vi "HFRR ADV v013 new software.vi"() -> ()   [LabVIEW 2025] (continued)
            n3539 = property class="DigNum (strict)"("Numeric Text.Text Colors:Text Color"="NI Text  2") -> ()  [unwired: 2 in, 2 out]
            n3540 = property class="DigNum (strict)"("Numeric Text.Text Colors:Text Color"="NI Text  2") -> ()  [unwired: 2 in, 2 out]
            n3541 = property on="Coefficient Of Friction" class="XYGraph (strict)"("Plot Area:Colors:FG Color"="GFG  2", "Plot Area:Colors:BG Color"="GBG   2") -> ()  [unwired: 2 in, 2 out]
            n3542 = property on="Humidity ( %RH )" class="XYGraph (strict)"("Plot Area:Colors:FG Color"="GFG  2", "Plot Area:Colors:BG Color"="GBG   2") -> ()  [unwired: 2 in, 2 out]
            n3543 = property on="Air Temperature  ( °C )" class="XYGraph (strict)"("Plot Area:Colors:FG Color"="GFG  2", "Plot Area:Colors:BG Color"="GBG   2") -> ()  [unwired: 2 in, 2 out]
            n3544 = property on="Sample Temperature ( °C )" class="XYGraph (strict)"("Plot Area:Colors:FG Color"="GFG  2", "Plot Area:Colors:BG Color"="GBG   2") -> ()  [unwired: 2 in, 2 out]
            n3545 = property class="DigNum (strict)"("Numeric Text.Text Colors:BG Color"="NI BG 2") -> ()  [unwired: 2 in, 2 out]
            n3546 = property class="DigNum (strict)"("Numeric Text.Text Colors:BG Color"="NI BG 2") -> ()  [unwired: 2 in, 2 out]
            n3547 = property class="DigNum (strict)"("Numeric Text.Text Colors:BG Color"="NI BG 2") -> ()  [unwired: 2 in, 2 out]
            n3548 = property class="DigNum (strict)"("Numeric Text.Text Colors:BG Color"="NI BG 2") -> ()  [unwired: 2 in, 2 out]
            n3549 = property class="DigNum (strict)"("Numeric Text.Text Colors:BG Color"="NI BG 2") -> ()  [unwired: 2 in, 2 out]
            n3550 = property class="DigNum (strict)"("Numeric Text.Text Colors:BG Color"="NI BG 2") -> ()  [unwired: 2 in, 2 out]
            n3551 = property class="DigNum (strict)"("Numeric Text.Text Colors:BG Color"="NI BG 2") -> ()  [unwired: 2 in, 2 out]
            n3552 = property class="DigNum (strict)"("Numeric Text.Text Colors:BG Color"="NI BG 2") -> ()  [unwired: 2 in, 2 out]
            n3553 = property class="DigNum (strict)"("Numeric Text.Text Colors:BG Color"="NI BG 2") -> ()  [unwired: 2 in, 2 out]
            n3554 = property class="DigNum (strict)"("Numeric Text.Text Colors:BG Color"="NI BG 2") -> ()  [unwired: 2 in, 2 out]
            n3555 = property class="DigNum (strict)"("Numeric Text.Text Colors:BG Color"="NI BG 2") -> ()  [unwired: 2 in, 2 out]
            n3556 = property class="DigNum (strict)"("Numeric Text.Text Colors:BG Color"="NI BG 2") -> ()  [unwired: 2 in, 2 out]
            n3557 = property class="DigNum (strict)"("Numeric Text.Text Colors:BG Color"="NI BG 2") -> ()  [unwired: 2 in, 2 out]
            n3558 = property class="DigNum (strict)"("Numeric Text.Text Colors:BG Color"="NI BG 2") -> ()  [unwired: 2 in, 2 out]
            n3559 = property class="DigNum (strict)"("Numeric Text.Text Colors:BG Color"="NI BG 2") -> ()  [unwired: 2 in, 2 out]
            n3560 = property class="Bool"("Colors [4]"="Boolean BC T & BG") -> ()  [unwired: 2 in, 2 out]
            n3561 = property on="Save & Continue" class="Bool (strict)"("Colors [4]"="Boolean BC T & BG") -> ()  [unwired: 2 in, 2 out]
            n3562 = property on="Heater Button" class="Bool (strict)"("Colors [4]"="Boolean BC T & BG") -> ()  [unwired: 2 in, 2 out]
            n3563 = property class="Bool"("Colors [4]"="Boolean BC T & BG") -> ()  [unwired: 2 in, 2 out]
            n3564 = property on="Humidity" class="Bool (strict)"("Colors [4]"="Boolean BC T & BG") -> ()  [unwired: 2 in, 2 out]
            n3565 = property class="Bool (strict)"("Colors [4]"="Boolean BC T & BG") -> ()  [unwired: 2 in, 2 out]
            n3566 = property on="RUN" class="Bool (strict)"("Colors [4]"="Boolean BC T & BG") -> ()  [unwired: 2 in, 2 out]
            n3567 = property on="trip1 8" class="Bool (strict)"("Colors [4]"="Boolean BC T & BG") -> ()  [unwired: 2 in, 2 out]
            n3568 = property class="Bool"("Colors [4]"="Boolean BC T & BG") -> ()  [unwired: 2 in, 2 out]
            n3569 = property class="Bool (strict)"("Colors [4]"="Boolean BC T & BG") -> ()  [unwired: 2 in, 2 out]
            n3570 = property on="OPEN 1" class="Bool (strict)"("Colors [4]"="Boolean BC T & BG 2") -> ()  [unwired: 2 in, 2 out]
            n3571 = property on="OPEN 2" class="Bool (strict)"("Colors [4]"="Boolean BC T & BG 2") -> ()  [unwired: 2 in, 2 out]
            n3572 = property on="OPEN 3" class="Bool (strict)"("Colors [4]"="Boolean BC T & BG 2") -> ()  [unwired: 2 in, 2 out]
            n3573 = property on="OPEN 4" class="Bool (strict)"("Colors [4]"="Boolean BC T & BG 2") -> ()  [unwired: 2 in, 2 out]
            n3574 = property on="OPEN" class="Bool (strict)"("Colors [4]"="Boolean BC T & BG 2") -> ()  [unwired: 2 in, 2 out]
            n3575 = property on="rstv2" class="Bool"("Colors [4]"="Boolean BC T & BG 2") -> ()  [unwired: 2 in, 2 out]
            n3576 = property on="RST CP" class="Bool"("Colors [4]"="Boolean BC T & BG 2") -> ()  [unwired: 2 in, 2 out]
            n3577 = property on="RSTV1 3" class="Bool"("Colors [4]"="Boolean BC T & BG 2") -> ()  [unwired: 2 in, 2 out]
            n3578 = property on="RSTV1 2" class="Bool"("Colors [4]"="Boolean BC T & BG 2") -> ()  [unwired: 2 in, 2 out]
          }
          frame #1 {
          }
        }
        n3579 = local read "Quit"() -> (w4455:bool)
      }
    }
    frame Enabled {
    }
  }
  n3580 = while {
    shift-right: [w4473] -> _
    shift-left: _ -> [w4474]
    shift-right: [w4471] -> _
    shift-left: T18 {"Read Heave and Surge"="", "Bytes at Heave Port"=0.0, "Heave and Surge COM Port:"="COM9", "Com Port 2"="COM7", "Residual Due"="", "Heave COM Status 2"=TRUE, "Heave COM Status"=TRUE, "Port 2"=TRUE, "Sway PPR"=6400.0, "Surge PPR"=6400.0, "Heave PPR"=6400.0, "Sway Pitch"=2.0, "Surge Pitch"=3.0, "Heave Pitch"=4.0, "Sway Pulses/mm"=320.0, "Surge Pulses/mm"=1600.0, "Heave Pulses/mm"=1600.0, "inner loop"=0.0, "Read Heave and Surge 2"="", "String 36"="", "Write S"=FALSE, "WriteCC1"=[""], "Heave COM Loop"=0, "LastCom"="", "EXIT"=FALSE, "Error Heave"={"status"=TRUE, "code"=-1073807343, "source"=""}} -> [w4470]
    shift-right: [w4468] -> _
    shift-left: enum16{"init", "MAIN", "Panel Close"}."init" -> [w4469]
    stop <- w4472 stop-if-true
    n3581 = case shown="\"MAIN\"" w4469 {
      tunnel: w4474 -> [w4488 w4503 w4564 w4566]
      tunnel: [w4482 w4512 w4564 w4566] -> w4473
      tunnel: [_ _ TRUE _] -> w4472
      tunnel: [w4478 w4509 w4562 w4565] -> w4471
      tunnel: w4470 -> [w4485 w4502 w4562 w4565]
      tunnel: [enum16{"init", "MAIN", "Panel Close"}."MAIN" w4496 _ _] -> w4468
      frame "init" {
        n3582 = Bundle By Name(cluster=w4485, "Heave and Surge COM Port:"="C3 :") -> (w4484:T18)
        n3583 = call "Instrument fgv.vi"("Enum"=T30."INIT", "error in (no error) 2"=w4488, "INPUT"=w4484) -> ("error"=w4486:errorcluster, "output"=w4481:T18)  [unwired: 6 in, 1 out]
        n3584 = case shown="Error" w4486 {
          selector: w4486 -> [w4490 _]
          tunnel: [w4490 w4494] -> w4482
          tunnel: w4481 -> [w4489 w4492]
          tunnel: [w4489 w4491] -> w4479
          frame No Error {
          }
          frame Error {
            n3585 = call "Instrument fgv.vi"("Enum"=T30."ERROR INIT", "INPUT"=w4492) -> ("error"=w4495:errorcluster, "output"=w4491:T18)  [unwired: 7 in, 1 out]
            n3586 = call <vilib>:"Clear Errors.vi"("error in (no error)"=w4495) -> ("error out"=w4494:errorcluster)  [unwired: 5 in, 1 out]
          }
        }
        n3587 = local read "LastCom"() -> (w4477:string)
        n3588 = Unbundle By Name(w4479) -> ("Heave COM Status 2"=→"COM Status" →"Instrument Status":bool, "Error Heave"=→"Error":errorcluster)  [unwired: 1 out]
        n3589 = Bundle By Name(cluster=w4479, "LastCom"=w4477) -> (w4478:T18)
      }
      frame "MAIN" {
        n3590 = Unbundle By Name(w4502) -> ("Com Port 2"=w4514:refnum<visa-resource-name>)
        n3591 = local write "Com Port 4"(w4514) -> ()
        n3592 = local read "C3 :"() -> (w4500:refnum<visa-resource-name>)
        n3593 = Bundle By Name(cluster=w4502, "Heave and Surge COM Port:"=w4500) -> (w4501:T18)
        n3594 = Equal?(x=w4514, y=w4500) -> (x = y?=w4513:bool)
        n3595 = case shown="True" w4513 {
          tunnel: [w4518 w4535] -> w4512
          tunnel: w4503 -> [w4519 w4541]
          tunnel: w4501 -> [w4517 w4539]
          tunnel: [w4516 w4534] -> w4509
          frame False {
            n3596 = call <vilib>:"Clear Errors.vi"("error in (no error)"=w4519) -> ("error out"=w4515:errorcluster)  [unwired: 5 in, 1 out]
            n3597 = call "Instrument fgv.vi"("Enum"=T30."ERROR INIT", "error in (no error) 2"=w4515, "INPUT"=w4517) -> ("error"=w4521:errorcluster, "output"=w4516:T18)  [unwired: 6 in, 1 out]
            n3598 = call <vilib>:"Clear Errors.vi"("error in (no error)"=w4521) -> ("error out"=w4518:errorcluster)  [unwired: 5 in, 1 out]
          }
          frame True {
            n3599 = call "Instrument fgv.vi"("Enum"=T30."READ", "error in (no error) 2"=w4541, "INPUT"=w4539) -> ("error"=w4540:errorcluster, "output"=w4531:T18)  [unwired: 6 in, 1 out]
            n3600 = Bundle By Name(cluster=w4531, "String 36"="String 11") -> (w4530:T18)
            n3601 = case shown="True" "Write S" {
              selector: "Write S" -> [_ w4561]
              tunnel: w4540 -> [w4554 w4560]
              tunnel: [w4554 w4559] -> w4527
              tunnel: w4530 -> [w4553 w4556]
              tunnel: [w4553 w4555] -> w4526
              frame False {
              }
              frame True {
                n3602 = Not(x=w4561) -> (.not. x?=w4557:bool)
                n3603 = local write "Write S"(w4557) -> ()
                n3604 = call "Instrument fgv.vi"("Enum"=T30."MANUAL WRITE", "error in (no error) 2"=w4560, "INPUT"=w4556) -> ("error"=w4559:errorcluster, "output"=w4555:T18)  [unwired: 6 in, 1 out]
              }
            }
            n3605 = Array Size(array="WriteHumidity") -> (size(s)=w4524:i32)
            n3606 = Greater Than 0?(x=w4524) -> (x > 0?=w4522:bool)
            n3607 = call "Instrument fgv.vi"("Enum"=T30."WRITE", "error in (no error) 2"=w4527, "WriteCC1"="WriteHumidity", "INPUT"=w4526) -> ("error"=w4537:errorcluster, "WriteCC1 2"=w4525:string[], "output"=w4536:T18)  [unwired: 5 in]
            n3608 = case shown="True" w4522 {
              tunnel: w4525 -> [_ w4543]
              frame False {
              }
              frame True {
                n3609 = local write "WriteHumidity"(w4543) -> ()
              }
            }
            n3610 = case shown="Error" w4537 {
              selector: w4537 -> [w4544 w4547]
              tunnel: w4536 -> [w4545 w4552]
              tunnel: [w4545 w4551] -> w4534
              tunnel: [w4544 w4549] -> w4535
              frame No Error {
              }
              frame Error {
                n3611 = call <vilib>:"Clear Errors.vi"("error in (no error)"=w4547) -> ("error out"=w4546:errorcluster)  [unwired: 5 in, 1 out]
                n3612 = call "Instrument fgv.vi"("Enum"=T30."ERROR INIT", "error in (no error) 2"=w4546, "INPUT"=w4552) -> ("error"=w4550:errorcluster, "output"=w4551:T18)  [unwired: 6 in, 1 out]
                n3613 = call <vilib>:"Clear Errors.vi"("error in (no error)"=w4550) -> ("error out"=w4549:errorcluster)  [unwired: 5 in, 1 out]
              }
            }
            n3614 = Unbundle By Name(w4534) -> ("LastCom"=→"LastCom":string, "Read Heave and Surge"=→"Read Humidity":string)
          }
        }
        n3615 = Unbundle By Name(w4509) -> ("Heave COM Status 2"=w4511:bool, "Heave COM Status"=w4510:bool, "Error Heave"=w4507:errorcluster, "Bytes at Heave Port"=→"Bytes at Humidity Port":dbl)
        n3616 = Unbundle By Name(w4507) -> ("status"=→"Humidity Port":bool)
        n3617 = Not(x=w4510) -> (.not. x?=w4504:bool)
        n3618 = local write "Error"(w4507) -> ()
        n3619 = Not(x=w4511) -> (.not. x?=w4505:bool)
        n3620 = local write "Instrument Status"(w4504) -> ()
        n3621 = local write "COM Status"(w4505) -> ()
        n3622 = local read "Quit"() -> (w4497:bool)
        n3623 = Select(t=enum16{"init", "MAIN", "Panel Close"}."Panel Close", s=w4497, f=enum16{"init", "MAIN", "Panel Close"}."MAIN") -> (s? t:f=w4496:enum16{"init", "MAIN", "Panel Close"})
      }
      frame "Panel Close" {
      }
      frame Default {
      }
    }
  }
  n3624 = while {
    stop <- w4592 stop-if-true
    n3625 = local read "Read Humidity"() -> (w4573:string)
    n3626 = call <vilib>:"High Resolution Polling Wait.vi"("seconds to wait"=0.1) -> ()  [unwired: 10 in, 1 out]
    n3627 = Spreadsheet String To Array(delimiter (Tab)=",", format string="", spreadsheet string=w4573, array type (2D Dbl)=string[] []) -> (array=w4587:string[])
    n3628 = for {
      tunnel: w4587 -> [w4597] mode=indexing
      tunnel: string[] ["STATE;", "SET;", "RH;", "T;", "AMB_RH;", "AMB_T;", "PUMP;", "FAN_IN;", "FAN_OUT;", "DEHUM;", "CURRENT;", "STALL;"] -> [w4596] mode=indexing
      tunnel: [w4595] -> w4586 mode=indexing
      n3629 = Match Pattern(string=w4597, regular expression=w4596) -> (after substring=w4595:string)  [unwired: 1 in, 3 out]
    }
    n3630 = Index Array(array=w4586) -> (element #1=→"STATE :":string, element #2=→"SET :":string, element #3=w4575:string, element #4=→"T :":string, element #5=w4572:string, element #6=→"AMB_T :":string, element #7=→"PUMP :":string, element #8=→"FAN_IN :":string, element #9=→"FAN_OUT :":string, element #10=→"DEHUM :":string, element #11=→"CURRENT :":string, element #12=→"STALL :":string)  [unwired: 12 in]
    "RH :" <- w4575
    "AMB_RH :" <- w4572
    n3631 = Fract/Exp String To Number(string=w4575) -> (number=w4567:dbl)  [unwired: 3 in, 1 out]
    n3632 = Fract/Exp String To Number(string=w4572) -> (number=w4571:dbl)  [unwired: 3 in, 1 out]
    n3633 = local write "Ambient Humidity :"(w4571) -> ()
    n3634 = Equal?(x=w4567, y=0.0) -> (x = y?=w4569:bool)
    n3635 = case shown="True" w4569 {
      tunnel: [w4593 w4594] -> w4568
      tunnel: w4567 -> [w4593 _]
      frame False {
        (unwired) 0.0
        "Humidity temp" <- w4593
      }
      frame True {
        n3636 = local read "Humidity temp"() -> (w4594:dbl)
      }
    }
    "RH Numeric:" <- w4568
    n3637 = local read "Quit"() -> (w4592:bool)
  }
  n3638 = disable-structure shown="Disabled" {
    frame Disabled {
      n3639 = while {
        tunnel: [w4831] -> _
        i -> [w4831]
        stop <- w4828 stop-if-true
        n3640 = local read "powstat"() -> (w4829:bool)
        n3641 = case shown="True" w4829 {
          frame False {
          }
          frame True {
            n3642 = local read "RUN"() -> (w4832:bool)
            n3643 = case shown="True" w4832 {
              frame False {
                w4862 = 65.0 ("y")
                n3644 = local read "Set Hz"() -> (w4890:dbl)
                n3645 = local read "NORMAL LOAD"() -> (w4891:dbl)
                n3646 = Multiply(x=w4890, y=60.0) -> (x*y=w4897:dbl)
                n3647 = Multiply(x=1.2 ("y"), y=0.949) -> (x*y=w4866:dbl)
                n3648 = Multiply(x=1.2 ("y"), y=0.8166) -> (x*y=w4870:dbl)
                n3649 = Multiply(x=1.2 ("y"), y=0.851) -> (x*y=w4865:dbl)
                n3650 = local read "FF 2"() -> (w4889:dbl)
                n3651 = Absolute Value(x=w4897) -> (abs(x)=w4895:dbl)
                n3652 = case shown="13.." w4889 {
                  tunnel: [1 2 3] -> w4887
                  frame 0..10, Default {
                    # "Normal"
                  }
                  frame 11, 12 {
                  }
                  frame 13.. {
                  }
                }
                "FF STATE" <- w4887
                n3653 = local read "TEMP"() -> (w4850:dbl)
                n3654 = local read item#-1() -> (w4864)
                n3655 = Less?(x=w4864, y=w4870) -> (x < y?=w4867:bool)
                n3656 = In Range and Coerce(upper limit=w4866, x=w4864, lower limit=w4865) -> (In Range?=w4868:bool)  [unwired: 1 out]
                n3657 = case shown="3601.." w4895 {
                  tunnel: [1 2 3] -> w4893
                  frame 0..3000, Default {
                    # "Normal"
                  }
                  frame 3001..3600 {
                  }
                  frame 3601.. {
                  }
                }
                n3658 = case shown="11.." w4891 {
                  tunnel: [1 3] -> w4892
                  frame 1..10, Default {
                  }
                  frame 11.. {
                  }
                }
                "NL STATE" <- w4892
                n3659 = Multiply(x=1.2 ("y"), y=0.95) -> (x*y=w4880:dbl)
                n3660 = Multiply(x=w4862, y=0.954) -> (x*y=w4854:dbl)
                n3661 = Or(x=w4867, y=w4868) -> (x .or. y?=w4869:bool)
                n3662 = Greater Or Equal?(x=w4864, y=w4880) -> (x >= y?=w4877:bool)
                n3663 = Multiply(x=w4862, y=0.99) -> (x*y=w4851:dbl)
                n3664 = Greater Or Equal?(x=w4850, y=w4851) -> (x >= y?=w4856:bool)
                n3665 = Greater Or Equal?(x=w4850, y=w4854) -> (x >= y?=w4853:bool)
                n3666 = case shown="0, 1, Default" w4864 {
                  tunnel: [1 3] -> w4881
                  frame 0, 1, Default {
                  }
                  frame 2.. {
                  }
                }
                n3667 = case shown="True" w4877 {
                  tunnel: [1 3] -> w4882
                  frame False {
                  }
                  frame True {
                  }
                }
                n3668 = case shown="True" w4869 {
                  tunnel: [1 2] -> w4883
                  frame False {
                  }
                  frame True {
                  }
                }
                n3669 = case shown="..0" w4850 {
                  tunnel: [2 3 3 1] -> w4857
                  frame 61, 62 {
                  }
                  frame 63.. {
                  }
                  frame ..0 {
                  }
                  frame 10..60, Default {
                  }
                }
                n3670 = case shown="True" w4856 {
                  tunnel: [1 3] -> w4858
                  frame False {
                  }
                  frame True {
                  }
                }
                n3671 = Number To Decimal String(number=w4893) -> (decimal integer string=w4894:string)  [unwired: 1 in]
                n3672 = case shown="True" w4853 {
                  tunnel: [1 2] -> w4859
                  frame False {
                  }
                  frame True {
                  }
                }
                n3673 = Number To Decimal String(number=1) -> (decimal integer string=→"Air temp":string)  [unwired: 1 in]
                n3674 = Number To Decimal String(number=w4887) -> (decimal integer string=→"ff_st":string)  [unwired: 1 in]
                n3675 = local write "sp_st"(w4894) -> ()
                n3676 = Number To Decimal String(number=w4892) -> (decimal integer string=→"nl_st":string)  [unwired: 1 in]
                n3677 = Build Array(w4857, w4858, w4859) -> (w4860:i32[])
                n3678 = Build Array(w4881, w4882, w4883) -> (w4884:i32[])
                n3679 = Array Max & Min(array=w4860) -> (max value=w4861:i32)  [unwired: 3 out]
                n3680 = Array Max & Min(array=w4884) -> (max value=w4885:i32)  [unwired: 3 out]
                n3681 = Number To Decimal String(number=w4861) -> (decimal integer string=w4849:string)  [unwired: 1 in]
                n3682 = Number To Decimal String(number=w4885) -> (decimal integer string=→"Stroke Ln 2":string)  [unwired: 1 in]
                n3683 = local write "temp_st"(w4849) -> ()
              }
              frame True {
                w4947 = 65.0 ("y")
                # "Healthy -1\nWarning -2\nError -3"
                n3684 = local read "TEMP"() -> (w4958:dbl)
                n3685 = local read "NORMAL LOAD"() -> (w4962:dbl)
                n3686 = local read "Set Hz"() -> (w4960:dbl)
                n3687 = Multiply(x=1.2 ("y"), y=0.949) -> (x*y=w4942:dbl)
                n3688 = Multiply(x=1.2 ("y"), y=0.8166) -> (x*y=w4938:dbl)
                n3689 = Multiply(x=1.2 ("y"), y=0.851) -> (x*y=w4943:dbl)
                n3690 = Multiply(x=w4947, y=0.954) -> (x*y=w4954:dbl)
                n3691 = Multiply(x=w4947, y=0.99) -> (x*y=w4957:dbl)
                n3692 = Greater Or Equal?(x=w4958, y=w4957) -> (x >= y?=w4952:bool)
                n3693 = Multiply(x=w4960, y=60.0) -> (x*y=w4966:dbl)
                n3694 = Greater Or Equal?(x=w4958, y=w4954) -> (x >= y?=w4955:bool)
                n3695 = local read "FF 2"() -> (w4961:dbl)
                n3696 = local read item#-1() -> (w4944)
                n3697 = Less?(x=w4944, y=w4938) -> (x < y?=w4941:bool)
                n3698 = In Range and Coerce(upper limit=w4942, x=w4944, lower limit=w4943) -> (In Range?=w4940:bool)  [unwired: 1 out]
                n3699 = Absolute Value(x=w4966) -> (abs(x)=w4964:dbl)
                n3700 = case shown="63.." w4958 {
                  tunnel: [2 3 3 1] -> w4951
                  frame 61, 62 {
                  }
                  frame 63.. {
                  }
                  frame ..0 {
                  }
                  frame 10..60, Default {
                  }
                }
                n3701 = case shown="True" w4952 {
                  tunnel: [1 3] -> w4950
                  frame False {
                  }
                  frame True {
                  }
                }
                n3702 = case shown="True" w4955 {
                  tunnel: [1 2] -> w4949
                  frame False {
                  }
                  frame True {
                  }
                }
                n3703 = Multiply(x=1.2 ("y"), y=0.95) -> (x*y=w4928:dbl)
                n3704 = case shown="1..10, Default" w4962 {
                  tunnel: [1 3] -> w4969
                  frame 1..10, Default {
                  }
                  frame 11.. {
                  }
                }
                n3705 = case shown="0..10, Default" w4961 {
                  tunnel: [1 2 3] -> w4968
                  frame 0..10, Default {
                  }
                  frame 11, 12 {
                  }
                  frame 13.. {
                  }
                }
                n3706 = case shown="3601.." w4964 {
                  tunnel: [1 2 3] -> w4963
                  frame 0..3000, Default {
                    # "Normal"
                  }
                  frame 3001..3600 {
                  }
                  frame 3601.. {
                  }
                }
                n3707 = Or(x=w4941, y=w4940) -> (x .or. y?=w4939:bool)
                n3708 = Greater Or Equal?(x=w4944, y=w4928) -> (x >= y?=w4931:bool)
                n3709 = case shown="0, 1, Default" w4944 {
                  tunnel: [1 3] -> w4927
                  frame 0, 1, Default {
                  }
                  frame 2.. {
                  }
                }
                n3710 = case shown="True" w4931 {
                  tunnel: [1 3] -> w4926
                  frame False {
                  }
                  frame True {
                  }
                }
                n3711 = case shown="True" w4939 {
                  tunnel: [1 2] -> w4925
                  frame False {
                  }
                  frame True {
                  }
                }
                n3712 = Build Array(w4951, w4950, w4949) -> (w4948:i32[])
                n3713 = Number To Decimal String(number=w4963) -> (decimal integer string=→"sp_st":string)  [unwired: 1 in]
                n3714 = Array Max & Min(array=w4948) -> (max value=w4945:i32)  [unwired: 3 out]
                "TEMP STATE" <- w4945
                n3715 = Number To Decimal String(number=w4969) -> (decimal integer string=w4972:string)  [unwired: 1 in]
                n3716 = Number To Decimal String(number=w4968) -> (decimal integer string=w4970:string)  [unwired: 1 in]
                n3717 = Number To Decimal String(number=w4945) -> (decimal integer string=→"temp_st":string)  [unwired: 1 in]
                n3718 = Build Array(w4927, w4926, w4925) -> (w4924:i32[])
                n3719 = local write "nl_st"(w4972) -> ()
                n3720 = local write "ff_st"(w4970) -> ()
                n3721 = Number To Decimal String(number=1) -> (decimal integer string=w4967:string)  [unwired: 1 in]
                n3722 = Array Max & Min(array=w4924) -> (max value=w4923:i32)  [unwired: 3 out]
                n3723 = local write "Air temp"(w4967) -> ()
                n3724 = Number To Decimal String(number=w4923) -> (decimal integer string=w4922:string)  [unwired: 1 in]
                n3725 = local write "Stroke Ln 2"(w4922) -> ()
              }
            }
            n3726 = local read "Stroke Ln 2"() -> (w4834:string)
            n3727 = local read "nl_st"() -> (w4840:string)
            n3728 = local read "ff_st"() -> (w4837:string)
            n3729 = local read "sp_st"() -> (w4838:string)
            n3730 = local read "temp_st"() -> (w4839:string)
            n3731 = local read "Air temp"() -> (w4833:string)
            n3732 = Replace Array Subset(array="in", new element #1=w4840, index #1=1 ("index"), new element #2=w4837, index #2=2 ("index"), new element #3=w4839, index #3=3 ("index"), new element #4=w4838, index #4=4 ("index"), new element #5=w4834, index #5=5 ("index"), new element #6=w4833, index #6=6 ("index"), new element #7="Sensor State" ("new element/subarray"), index #7=0 ("index")) -> (→"out":string[])
          }
        }
        n3733 = Wait (ms)(milliseconds to wait=u32 10) -> ()  [unwired: 1 out]
        n3734 = local read "Quit"() -> (w4828:bool)
      }
      n3735 = while {
        stop <- w4803 stop-if-true
        n3736 = local read "run replace"() -> (w4805:bool)
        n3737 = Wait (ms)(milliseconds to wait=u32 100) -> ()  [unwired: 1 out]
        n3738 = Equal?(x="FLAG 2", y=0.0) -> (x = y?=w4806:bool)
        n3739 = case shown="True" w4806 {
          frame False {
          }
          frame True {
            n3740 = local write "FLAG 2"(100.0 ("FLAG 2")) -> ()
            n3741 = call <vilib>:"Read Characters From File.vi"("file path (dialog if empty)"=path "C:/LAB-IQ-NXT/WO 2449 TT.sig", "convert eol? (no:F)"=FALSE ("append to file? (new file:F)")) -> ("character string"=w4809:string)  [unwired: 4 in, 3 out]
            n3742 = call <vilib>:"Read Characters From File.vi"("file path (dialog if empty)"=path "C:/LAB-IQ-NXT/WO 2449 TRH.sig", "convert eol? (no:F)"=FALSE ("append to file? (new file:F)")) -> ("character string"=w4810:string)  [unwired: 4 in, 3 out]
            n3743 = Decimal String To Number(string=w4809) -> (number=w4811:i32)  [unwired: 2 in, 1 out]
            n3744 = local write "Total No. of Tests"(w4811) -> ()
            n3745 = Decimal String To Number(string=w4810) -> (number=w4814:i32)  [unwired: 2 in, 1 out]
            n3746 = local write "SEN.RUN HRS"(w4814) -> ()
          }
        }
        n3747 = case shown="True" w4805 {
          frame False {
          }
          frame True {
            n3748 = Equal?(x="FLAG 4", y=0.0) -> (x = y?=w4818:bool)
            n3749 = case shown="False" w4818 {
              frame False {
                n3750 = Get Date/Time In Seconds() -> (seconds since 1Jan1904=w4824:timestamp)
                n3751 = local read "START 3"() -> (w4822:dbl)
                n3752 = To Double Precision Float(number=w4824) -> (double precision float=w4823:dbl)
                n3753 = Subtract(x=w4823, y=w4822) -> (x-y=→"SENSOR TIME":dbl)
              }
              frame True {
                n3754 = Get Date/Time In Seconds() -> (seconds since 1Jan1904=w4826:timestamp)
                n3755 = local write "FLAG 4"(100.0 ("FLAG")) -> ()
                n3756 = To Double Precision Float(number=w4826) -> (double precision float=→"START 3":dbl)
              }
            }
          }
        }
        n3757 = local read "Quit"() -> (w4803:bool)
      }
      n3758 = while {
        shift-right: [w4603] -> _
        shift-left: _ -> [w4604]
        tunnel: [w4599] -> _
        i -> [w4599]
        stop <- w4598 stop-if-true
        n3759 = Wait (ms)(milliseconds to wait=u32 50 ("Refresh Rate (ms)")) -> ()  [unwired: 1 out]
        n3760 = local read "Json End Flg"() -> (w4600:bool)
        n3761 = Not(x="Upld AR 2") -> ()  [unwired: 1 out]
        n3762 = local read "Upld AR 2"() -> (w4601:bool)
        n3763 = call "Elapsed Time9"("Time Target (s)"="Sen.Upload Rate (s)", "Reset"=FALSE, "Auto Reset"=TRUE) -> ("Time has Elapsed"=w4610:bool)  [unwired: 9 in, 7 out]
        n3764 = Or(x=w4610, y=w4600) -> (x .or. y?=w4606:bool)
        n3765 = case shown="True" w4606 {
          frame False {
          }
          frame True {
            w4702 = "\"SensorName\":\"" ("string")
            w4672 = " \"},{"
            w4697 = "\",\"SensorState\":\""
            w4699 = "\",\"SensorModelNumber\":\"" ("string")
            w4698 = "\",\"SensorRuntimeHours\":\"" ("string")
            n3766 = local read "model num"() -> (w4696:string[])
            n3767 = local read "Sensor name"() -> (w4715:string[])
            n3768 = local read "run"() -> (w4686:string[])
            n3769 = local read "SENSOR TIME"() -> (w4642:dbl)
            n3770 = local read "out"() -> (w4635:string[])
            n3771 = local read "Total No. of Tests"() -> (w4640:dbl)
            n3772 = Select(t=60.0, s="Run test 3", f=3600.0) -> (s? t:f=w4650:dbl)
            n3773 = Index Array(array=w4696, index #1=1 ("index")) -> (element #1=w4695:string, element #2=w4694:string, element #3=w4693:string, element #4=w4692:string, element #5=w4691:string, element #6=w4690:string)  [unwired: 5 in]
            n3774 = Index Array(array=w4686, index #1=1 ("index")) -> (element #1=w4685:string, element #2=w4684:string, element #3=w4683:string, element #4=w4682:string, element #5=w4681:string, element #6=w4680:string)  [unwired: 5 in]
            n3775 = Index Array(array=w4715, index #1=1 ("index")) -> (element #1=w4714:string, element #2=w4713:string, element #3=w4712:string, element #4=w4711:string, element #5=w4701:string, element #6=w4700:string)  [unwired: 5 in]
            n3776 = Index Array(array=w4635, index #1=1 ("index")) -> (element #1=w4667:string, element #2=w4666:string, element #3=w4665:string, element #4=w4664:string, element #5=w4663:string, element #6=w4662:string)  [unwired: 5 in]
            n3777 = local read "SEN.RUN HRS"() -> (w4638:dbl)
            n3778 = Divide(x=w4642, y=w4650) -> (x/y=w4649:dbl)
            n3779 = Increment(x=w4649) -> (x+1=w4645:dbl)
            n3780 = Number To Decimal String(number=w4645) -> (decimal integer string=→"run hrs":string)  [unwired: 1 in]
            n3781 = Divide(x=w4638, y=3600.0 ("f")) -> (x/y=w4633:dbl)
            n3782 = Round To Nearest(number=w4633) -> (nearest integer value=w4631:dbl)
            n3783 = Number To Decimal String(number=w4631) -> (decimal integer string=w4632:string)  [unwired: 1 in]
            n3784 = Number To Decimal String(number=w4640) -> (decimal integer string=w4641:string)  [unwired: 1 in]
            n3785 = local read "Model No"() -> (w4646:string)
            n3786 = local read "UUID"() -> (w4741:string)
            n3787 = local read "Serial No"() -> (w4745:string)
            n3788 = local read "Secret Key"() -> (w4746:string)
            n3789 = Concatenate Strings("\",\"MachineSerialNumber\":\"" ("string"), w4745) -> (w4749:string)
            n3790 = Concatenate Strings("\",\"ModelNumber\":\"" ("string"), w4646) -> (w4647:string)
            n3791 = Concatenate Strings("\",\"MachineRuntimeHours\":\"" ("string"), w4632) -> (w4750:string)
            n3792 = Concatenate Strings("\",\"MachineRuntimeCycles\":\"", w4641) -> (w4743:string)
            n3793 = Concatenate Strings(w4699, w4695) -> (w4729:string)
            n3794 = Concatenate Strings(w4698, w4685) -> (w4730:string)
            n3795 = Concatenate Strings(w4697, w4667) -> (w4728:string)
            n3796 = Concatenate Strings(w4749, w4647, w4750, w4743) -> (w4752:string)
            n3797 = Concatenate Strings(w4699, w4694) -> (w4726:string)
            n3798 = Concatenate Strings(w4698, w4684) -> (w4725:string)
            n3799 = Concatenate Strings(w4697, w4666) -> (w4727:string)
            n3800 = Concatenate Strings(w4699, w4693) -> (w4721:string)
            n3801 = Concatenate Strings(w4698, w4683) -> (w4722:string)
            n3802 = Concatenate Strings(w4697, w4665) -> (w4720:string)
            n3803 = Concatenate Strings(w4699, w4692) -> (w4718:string)
            n3804 = Concatenate Strings(w4698, w4682) -> (w4717:string)
            n3805 = Concatenate Strings(w4697, w4664) -> (w4719:string)
            n3806 = Concatenate Strings(w4729, w4730, w4728) -> (w4731:string)
            n3807 = Concatenate Strings(w4699, w4691) -> (w4708:string)
            n3808 = Concatenate Strings(w4698, w4681) -> (w4709:string)
            n3809 = Concatenate Strings(w4699, w4690) -> (w4705:string)
            n3810 = Concatenate Strings(w4698, w4680) -> (w4704:string)
            n3811 = Concatenate Strings(w4697, w4663) -> (w4707:string)
            n3812 = Concatenate Strings(w4697, w4662) -> (w4706:string)
            n3813 = Concatenate Strings("{\"SecretKey\":\"", w4746, w4752, "\",\"UUID\" : \"", w4741, "\",\"SensorInformation\":", "[{" ("string")) -> (w4679:string)
            n3814 = Concatenate Strings(w4726, w4725, w4727) -> (w4724:string)
            n3815 = Concatenate Strings(w4721, w4722, w4720) -> (w4723:string)
            n3816 = Concatenate Strings(w4718, w4717, w4719) -> (w4716:string)
            n3817 = Concatenate Strings(w4708, w4709, w4707) -> (w4710:string)
            n3818 = Concatenate Strings(w4705, w4704, w4706) -> (w4703:string)
            n3819 = Concatenate Strings(w4702, w4714, w4731, w4672) -> (w4678:string)
            n3820 = Concatenate Strings(w4702, w4713, w4724, w4672) -> (w4677:string)
            n3821 = Concatenate Strings(w4702, w4712, w4723, w4672) -> (w4676:string)
            n3822 = Concatenate Strings(w4702, w4711, w4716, w4672) -> (w4675:string)
            n3823 = Concatenate Strings(w4702, w4701, w4710, w4672) -> (w4674:string)
            n3824 = Concatenate Strings(w4702, w4700, w4703, "\"}" ("string")) -> (w4673:string)
            n3825 = Concatenate Strings(w4679, w4678, w4677, w4676, w4675, w4674, w4673, "]}" ("string")) -> (w4670:string)
            n3826 = local read "SEN.RUN HRS"() -> (w4637:dbl)
            n3827 = disable-structure shown="Disabled" {
              frame Disabled {
                n3828 = local read "state"() -> (w4756:string[])
                n3829 = Delete From Array(array=w4756, index=0) -> (array with subset deleted=w4754:string[])  [unwired: 1 in, 1 out]
                n3830 = for {
                  N: 6 -> [_]
                  tunnel: w4754 -> [w4767] mode=indexing
                  tunnel: [w4766] -> w4753 mode=indexing
                  n3831 = Equal?(x=w4767, y="Warning") -> (x = y?=w4763:bool)
                  n3832 = Equal?(x=w4767, y="Healthy") -> (x = y?=w4760:bool)
                  n3833 = Select(t="2" ("y"), s=w4763, f="3" ("y")) -> (s? t:f=w4758:string)
                  n3834 = Select(t="1" ("y"), s=w4760, f=w4758) -> (s? t:f=w4766:string)
                }
                "state1" <- w4753
              }
              frame Enabled {
              }
            }
            n3835 = stacked-sequence {
              tunnel: w4670 -> [w4778 _ _]
              tunnel: [_ _ w4794] -> _
              frame #0 {
                (unwired) FALSE ("convert eol (F)")
                w4780 = enum16{"start", "end", "current"}."start" ("pos mode (0:2)")
                n3836 = local read "Path"() -> (w4774:path)
                n3837 = Path To String(path=w4774) -> (string=w4786:string)
                n3838 = Concatenate Strings(w4786, "\\", "Sensor File Name") -> (w4787:string)
                n3839 = local write "standard output 2"(" ") -> ()
                n3840 = String To Path(string=w4787) -> (path=w4777:path)
                n3841 = call <vilib>:"Open_Create_Replace File.vi"("advisory dialog? (display:T)"=FALSE, "function (open:0)"=T31."create or replace", "file path"=w4777) -> ("error out"=w4790:errorcluster, "refnum"=w4789:refnum<file>)  [unwired: 5 in, 2 out]
                n3842 = Set File Position(refnum=w4789, from (0:start)=w4780, error in=w4790) -> (refnum out=w4770:refnum<file>, error out=w4769:errorcluster)  [unwired: 1 in]
                n3843 = Write to Binary File(file (use dialog)=w4770, data=" ", error in=w4769, 5:FALSE ("prepend array or string size? (T)")) -> (refnum out=w4781:refnum<file>, error out=w4782:errorcluster)  [unwired: 2 in, 1 out]
                n3844 = Set File Position(offset (in bytes) (0)=w4780, refnum=w4781, error in=w4782) -> (refnum out=w4773:refnum<file>, error out=w4772:errorcluster)  [unwired: 1 in]
                n3845 = Write to Binary File(file (use dialog)=w4773, data=w4778, error in=w4772, 5:FALSE ("prepend array or string size? (T)")) -> (error out=w4776:errorcluster)  [unwired: 2 in, 2 out]
                n3846 = flat-sequence {
                  tunnel: w4777 -> [w4792]
                  tunnel: w4776 -> [_]
                  frame #0 {
                    n3847 = call <vilib>:"Read Characters From File.vi"("file path (dialog if empty)"=w4792) -> ("character string"=→"Sensor Health JSON string":string)  [unwired: 5 in, 3 out]
                  }
                }
                "SinglePoint  2" <- w4778
              }
              frame #1 {
              }
              frame #2 {
                (unwired) "\"Stored\": true" ("string")
                n3848 = call <vilib>:"System Exec.vi"("run minimized? (F)"=TRUE, "wait until completion? (T)"=TRUE, "working directory"=path "C:/LAB-IQ-NXT", "command line"="C:\\LAB-IQ-NXT\\JPostH.bat") -> ("standard error"=→"Respose From Server 2":string, "standard output"=w4797:string)  [unwired: 4 in, 2 out]
                "standard output 2" <- w4797
                n3849 = Match Pattern(string=w4797, regular expression="JSONH Check String") -> (match substring=w4795:string, offset past match=w4794:i32)  [unwired: 1 in, 2 out]
                n3850 = Equal?(x=w4795, y="JSONH Check String") -> (x = y?=→"Upload \nConfirmed 2":bool)
              }
            }
            n3851 = Divide(x=w4637, y=3600.0 ("f")) -> (x/y=w4630:dbl)
            n3852 = local read "run time"() -> (w4687:string[])
            n3853 = Round To Nearest(number=w4630) -> (nearest integer value=w4629:dbl)
            n3854 = Number To Decimal String(number=w4629) -> (decimal integer string=w4628:string)  [unwired: 1 in]
            n3855 = Index Array(array="Sensor Information", index (col) #1=0 ("disabled index (col)"), index (col) #2=1 ("index (col)"), index (col) #3=2 ("index (col)"), index (col) #4=3 ("index (col)")) -> (element #1=→"Sensor name":string[], element #2=→"model num":string[], element #3=→"run time":string[], element #4=→"state":string[])  [unwired: 4 in]
            n3856 = Insert Into Array(array=w4687, index=1, new element #1=w4628, new element #2=w4628, new element #3=w4628, new element #4=w4628, new element #5=w4628, new element #6=w4628) -> (w4652:string[])
            "run" <- w4652
            n3857 = local read "out"() -> (w4634:string[])
            n3858 = local read "Sensor Information"() -> (w4654:string[][])
            n3859 = Replace Array Subset(array=w4654, new element #1=w4652, index (col) #1=2 ("disabled index (col)"), new element #2=w4634, index (col) #2=3 ("index (col)")) -> (w4653:string[][])  [unwired: 2 in]
            n3860 = local write "Sensor Information"(w4653) -> ()
          }
        }
        n3861 = case shown="True" w4601 {
          frame False {
          }
          frame True {
            n3862 = Equal?(x="FLAG", y=0.0) -> (x = y?=w4618:bool)
            n3863 = case shown="False" w4618 {
              frame False {
                n3864 = Get Date/Time In Seconds() -> (seconds since 1Jan1904=w4624:timestamp)
                n3865 = local read "START 2"() -> (w4622:dbl)
                n3866 = To Double Precision Float(number=w4624) -> (double precision float=w4623:dbl)
                n3867 = Subtract(x=w4623, y=w4622) -> (x-y=→"SENSOR TIME  2":dbl)
              }
              frame True {
                n3868 = Get Date/Time In Seconds() -> (seconds since 1Jan1904=w4626:timestamp)
                n3869 = To Double Precision Float(number=w4626) -> (double precision float=→"START 2":dbl)
                n3870 = local write "FLAG"(100.0 ("FLAG")) -> ()
              }
            }
          }
        }
        n3871 = disable-structure shown="Disabled" {
          disable-tunnel: w4604 -> [w4613 _]
          disable-tunnel: [w4612 _] -> w4603
          frame Disabled {
            n3872 = local read "Json St Flg"() -> (w4611:bool)
            n3873 = case shown="True" w4611 {
              tunnel: w4613 -> [w4614 w4616]
              tunnel: [w4614 w4615] -> w4612
              frame False {
              }
              frame True {
                n3874 = Increment(x=w4616) -> (x+1=w4615:dbl)
                "T cycle" <- w4615
                n3875 = local write "Json St Flg"(FALSE ("Json St Flg")) -> ()
              }
            }
          }
          frame Enabled {
          }
        }
        n3876 = local read "Quit"() -> (w4598:bool)
      }
    }
    frame Enabled {
    }
  }
  n3877 = stacked-sequence {
    tunnel: [w4996] -> w38
    frame #0 {
      w4996 = FALSE ("Upload \nConfirmed")
      n3878 = local write "Upload \nConfirmed"(w4996) -> ()
      n3879 = local write "St Str"("") -> ()
    }
  }
  n3880 = disable-structure shown="Disabled" {
    disable-tunnel: w38 -> [w4997 _]
    frame Disabled {
      n3881 = case shown="True" {
        selector: _ -> [_ _]
        tunnel: w4997 -> [_ w4998]
        frame False {
        }
        frame True {
          n3882 = while {
            tunnel: [w5004] -> _
            tunnel: w4998 -> [_]
            i -> [w5004]
            stop <- w4999 stop-if-true
            n3883 = local read "Json End Flg"() -> (w5003:bool)
            n3884 = Wait (ms)(milliseconds to wait=u32 20 ("Refresh Rate (ms)")) -> ()  [unwired: 1 out]
            n3885 = local read "refresh flag"() -> (w5000:bool)
            n3886 = local read "RUN"() -> (w5001:bool)
            n3887 = And(x=w5001, y=w5000) -> (x .and. y?=w5002:bool)
            n3888 = Or(x=w5002, y=w5003) -> (x .or. y?=w5005:bool)
            "AR Led" <- w5005
            n3889 = case shown="True" w5005 {
              frame False {
              }
              frame True {
                w5022 = "\",\""
                n3890 = local read "UUID"() -> (w5020:string)
                n3891 = local write "refresh flag"(FALSE ("refresh flag")) -> ()
                n3892 = local read "time"() -> (w5009:dbl)
                n3893 = Multiply(x=w5009, y=60.0) -> (x*y=w5008:dbl)
                n3894 = Concatenate Strings("UUID\" : \"", w5020, "\"}") -> (w5023:string)
                n3895 = Number To Fractional String(number=w5008, width (-)=i16 10, precision (6)=i16 4) -> (F-format string=w5037:string)  [unwired: 1 in]
                n3896 = Concatenate Strings("{", "\"Time\":\"", w5037, w5022) -> (w5032:string)
                n3897 = stacked-sequence {
                  tunnel: w5022 -> [w5085 w5093 w5100 w5108 w5116 w5125 w5132]
                  tunnel: [w5086 _ _ _ _ _ _] -> w5036
                  tunnel: [_ w5094 _ _ _ _ _] -> w5035
                  tunnel: [_ _ w5101 _ _ _ _] -> w5034
                  tunnel: [_ _ _ w5110 _ _ _] -> w5033
                  tunnel: w5023 -> [_ _ _ _ _ _ w5143]
                  tunnel: [_ _ _ _ _ _ w5142] -> w5019
                  tunnel: [_ _ _ _ _ w5122 _] -> w5018
                  tunnel: [_ _ _ _ w5115 _ _] -> w5017
                  frame #0 {
                    n3898 = local read "NORMAL LOAD"() -> (w5084:dbl)
                    n3899 = Number To Fractional String(number=w5084, width (-)=i16 10, precision (6)=i16 4) -> (F-format string=w5087:string)  [unwired: 1 in]
                    n3900 = Concatenate Strings("NormalLoad\":\"", w5087, w5085) -> (w5086:string)
                  }
                  frame #1 {
                    n3901 = local read "Temp"() -> (w5092:dbl)
                    n3902 = Number To Fractional String(number=w5092, width (-)=i16 10, precision (6)=i16 4) -> (F-format string=w5095:string)  [unwired: 1 in]
                    n3903 = Concatenate Strings("Temperature\":\"", w5095, w5093) -> (w5094:string)
                  }
                  frame #2 {
                    n3904 = local read "cof"() -> (w5098:dbl)
                    n3905 = Number To Fractional String(number=w5098, width (-)=i16 10, precision (6)=i16 4) -> (F-format string=w5102:string)  [unwired: 1 in]
                    n3906 = Concatenate Strings("FrictionalForce\":\"", w5102, w5100) -> (w5101:string)
                  }
                  frame #3 {
                    n3907 = local read "Set Hz"() -> (w5106:dbl)
                    n3908 = Multiply(x=w5106, y=60.0) -> (x*y=w5105:dbl)
                    n3909 = Number To Fractional String(number=w5105, width (-)=i16 10, precision (6)=i16 4) -> (F-format string=w5111:string)  [unwired: 1 in]
                    n3910 = Concatenate Strings("Speed\":\"", w5111, w5108) -> (w5110:string)
                  }
                  frame #4 {
                    n3911 = local read item#-1() -> (w5114)
                    n3912 = Number To Fractional String(number=w5114, width (-)=i16 10, precision (6)=i16 4) -> (F-format string=w5118:string)  [unwired: 1 in]
                    n3913 = Concatenate Strings("LinearDeformation\":\"", w5118, w5116) -> (w5115:string)
                  }
                  frame #5 {
                    n3914 = local read "AIR TEMP"() -> (w5121:dbl)
                    n3915 = local read "Json St Flg"() -> (w5123:bool)
                    n3916 = local read "Json End Flg"() -> (w5124:bool)
                    n3917 = Number To Fractional String(number=w5121, width (-)=i16 10, precision (6)=i16 4) -> (F-format string=w5127:string)  [unwired: 1 in]
                    n3918 = Concatenate Strings("Vibration\":\"", w5127, w5125) -> (w5122:string)
                    n3919 = And(x=w5123, y=w5124) -> ()  [unwired: 1 out]
                  }
                  frame #6 {
                    n3920 = local read "Json End Flg"() -> (w5131:bool)
                    n3921 = Get Date/Time In Seconds() -> (seconds since 1Jan1904=w5139:timestamp)
                    n3922 = local read "Json St Flg"() -> (w5130:bool)
                    n3923 = To Double Precision Float(number=w5139) -> (double precision float=w5138:dbl)
                    n3924 = Subtract(x=w5138, y=2082844800.0) -> (x-y=w5136:dbl)
                    n3925 = Number To Fractional String(number=w5136, width (-)=i16 12, precision (6)=i16 0) -> (F-format string=w5133:string)  [unwired: 1 in]
                    n3926 = case shown="True" w5131 {
                      tunnel: ["" w5146] -> w5140
                      tunnel: w5133 -> [_ w5147]
                      tunnel: w5132 -> [_ w5145]
                      frame False {
                      }
                      frame True {
                        n3927 = local write "Json End Flg"(FALSE ("Json St Flg")) -> ()
                        n3928 = Concatenate Strings("End\": \"", w5147, w5145) -> (w5146:string)
                      }
                    }
                    n3929 = case shown="True" w5130 {
                      tunnel: [w5150 w5153] -> w5141
                      tunnel: w5133 -> [_ w5154]
                      tunnel: w5132 -> [_ w5151]
                      frame False {
                        n3930 = local read "St Str"() -> (w5150:string)
                      }
                      frame True {
                        n3931 = Concatenate Strings("Start\":\"", w5154, w5151) -> (w5153:string)
                        "St Str" <- w5153
                        n3932 = local write "Json St Flg"(FALSE ("Json St Flg")) -> ()
                      }
                    }
                    n3933 = Concatenate Strings(w5141, w5140, w5143) -> (w5142:string)
                  }
                }
                n3934 = local read "FILE"() -> (w5011:string)
                n3935 = Concatenate Strings("\",\"OperatorID\":\"" ("string"), "Operator ID") -> (w5014:string)
                n3936 = Concatenate Strings("\",\"DatasetTitle\":\"" ("string"), w5011) -> (w5013:string)
                n3937 = Concatenate Strings("\",\"SerialNumber\":\"" ("string"), "Serial No") -> (w5043:string)
                n3938 = Concatenate Strings("\",\"ModelNumber\":\"" ("string"), "Model No") -> (w5042:string)
                n3939 = Concatenate Strings(w5043, w5042) -> (w5025:string)
                n3940 = Concatenate Strings("{\"SecretKey\":\"", "Secret Key", w5025, w5014, w5013, "\",\"Samples\":[") -> (w5030:string)
                n3941 = Concatenate Strings(w5032, w5036, w5035, w5034, w5033, w5017, w5018, w5019) -> (w5031:string)
                n3942 = Concatenate Strings(w5030, w5031, "]}") -> (w5029:string)
                n3943 = stacked-sequence {
                  tunnel: w5029 -> [w5058 _ _]
                  tunnel: [_ _ w5075] -> _
                  frame #0 {
                    (unwired) FALSE ("convert eol (F)")
                    w5060 = enum16{"start", "end", "current"}."start" ("pos mode (0:2)")
                    n3944 = Path To String(path="Path") -> (string=w5066:string)
                    n3945 = Concatenate Strings(w5066, "\\", "Data File Name") -> (w5068:string)
                    n3946 = local write "standard output"(" ") -> ()
                    n3947 = String To Path(string=w5068) -> (path=w5057:path)
                    n3948 = call <vilib>:"Open_Create_Replace File.vi"("advisory dialog? (display:T)"=FALSE, "function (open:0)"=T31."create or replace", "file path"=w5057) -> ("error out"=w5071:errorcluster, "refnum"=w5070:refnum<file>)  [unwired: 5 in, 2 out]
                    n3949 = Set File Position(refnum=w5070, from (0:start)=w5060, error in=w5071) -> (refnum out=w5051:refnum<file>, error out=w5050:errorcluster)  [unwired: 1 in]
                    n3950 = Write to Binary File(file (use dialog)=w5051, data=" ", error in=w5050, 5:FALSE ("prepend array or string size? (T)")) -> (refnum out=w5061:refnum<file>, error out=w5062:errorcluster)  [unwired: 2 in, 1 out]
                    n3951 = Set File Position(offset (in bytes) (0)=w5060, refnum=w5061, error in=w5062) -> (refnum out=w5054:refnum<file>, error out=w5053:errorcluster)  [unwired: 1 in]
                    n3952 = Write to Binary File(file (use dialog)=w5054, data=w5058, error in=w5053, 5:FALSE ("prepend array or string size? (T)")) -> (error out=w5056:errorcluster)  [unwired: 2 in, 2 out]
                    n3953 = flat-sequence {
                      tunnel: w5057 -> [w5073]
                      tunnel: w5056 -> [_]
                      frame #0 {
                        n3954 = call <vilib>:"Read Characters From File.vi"("file path (dialog if empty)"=w5073) -> ("character string"=→"JSON string":string)  [unwired: 5 in, 3 out]
                      }
                    }
                    "SinglePoint" <- w5058
                  }
                  frame #1 {
                  }
                  frame #2 {
                    (unwired) "\"Stored\": true" ("string")
                    n3955 = call <vilib>:"System Exec.vi"("run minimized? (F)"=TRUE, "wait until completion? (T)"=TRUE, "working directory"=path "C:/LAB-IQ-NXT", "command line"="C:\\LAB-IQ-NXT\\JPost.bat") -> ("standard error"=→"Respose From Server":string, "standard output"=w5078:string)  [unwired: 4 in, 2 out]
                    "standard output" <- w5078
                    n3956 = Match Pattern(string=w5078, regular expression="JSON Check String") -> (match substring=w5076:string, offset past match=w5075:i32)  [unwired: 1 in, 2 out]
                    n3957 = Equal?(x=w5076, y="JSON Check String") -> (x = y?=→"Upload \nConfirmed":bool)
                  }
                }
              }
            }
            n3958 = local read "Quit"() -> (w4999:bool)
          }
        }
      }
    }
    frame Enabled {
    }
  }
  n3959 = disable-structure shown="Disabled" {
    disable-tunnel: _ -> [w5161 _]
    frame Disabled {
      n3960 = while {
        shift-right: [w5169] -> w5157
        shift-left: _ -> [w5170]
        shift-right: [w5167] -> w5158
        shift-left: errorcluster {"status"=TRUE, "code"=0, "source"="Init"} ("error out") -> [w5168]
        shift-right: [w5165] -> _
        shift-left: "" -> [w5166]
        tunnel: [w5163] -> _
        tunnel: w5161 -> [_]
        i -> [w5163]
        stop <- w5162 stop-if-true
        n3961 = flat-sequence {
          tunnel: [w5171] -> w5164
          frame #0 {
            n3962 = Wait (ms)(milliseconds to wait=10.0 ("Delay")) -> (millisecond timer value=w5171:u32)
          }
        }
        n3963 = case shown="No Error" w5168 {
          selector: w5168 -> [w5201 w5320]
          tunnel: [w5184 w5322] -> w5169
          tunnel: [w5183 w5321] -> w5167
          tunnel: w5170 -> [w5202 w5314]
          tunnel: w5166 -> [w5182 w5313]
          tunnel: [w5181 w5313] -> w5165
          tunnel: w5164 -> [_ _]
          frame No Error {
            n3964 = Concatenate Strings("\r", "\n") -> (w5193:string)  [unwired: 1 in]
            n3965 = case shown="True" w5194 {
              tunnel: w5202 -> [w5226 w5233]
              tunnel: w5201 -> [w5225 w5232]
              tunnel: [w5226 w5231] -> w5200
              tunnel: [w5225 w5230] -> w5180
              tunnel: w5193 -> [_ w5229]
              frame False {
              }
              frame True {
                n3966 = VISA Write(VISA resource name=w5233, write buffer=w5229, error in (no error)=w5232) -> (VISA resource name out=w5231:refnum<visa-resource-name>, error out=w5230:errorcluster)  [unwired: 1 out]
                n3967 = local write "Read String"("") -> ()
                n3968 = local write item#-1(FALSE) -> ()
              }
            }
            n3969 = property class="Instr"(reference=w5200, error in=w5180) -> (reference out=w5199:refnum<visa-resource-name>, error out=w5198:errorcluster, "Serial Settings:Number of Bytes at Serial Port"=w5197:u32)
            n3970 = Greater?(x=w5197, y=u32 100) -> (0:w5195:bool)
            n3971 = case shown="True" w5195 {
              tunnel: w5199 -> [w5236 w5260]
              tunnel: w5198 -> [w5235 w5259]
              tunnel: w5197 -> [_ w5258]
              tunnel: [w5236 w5257] -> w5186
              tunnel: [w5235 w5256] -> w5185
              tunnel: w5182 -> [w5234 w5255]
              tunnel: [w5234 ""] -> w5181
              frame False {
              }
              frame True {
                w5245 = u32 6 ("y")
                # "Page 84 of \nmanual"
                n3972 = VISA Read(VISA resource name=w5260, byte count=w5258, error in (no error)=w5259) -> (VISA resource name out=w5257:refnum<visa-resource-name>, read buffer=w5253:string, error out=w5256:errorcluster)  [unwired: 1 out]
                n3973 = while {
                  tunnel: w5253 -> [w5309]
                  tunnel: [w5305] -> w5247 mode=indexing
                  tunnel: [w5299] -> w5251 mode=indexing
                  tunnel: [w5297] -> _
                  i -> [w5297]
                  stop <- w5302 stop-if-true
                  n3974 = String Subset(string=w5309, offset (0)=w5297) -> (substring=w5304:string)  [unwired: 1 in]
                  n3975 = String To Byte Array(string=w5304) -> (unsigned byte array=w5308:u8[])
                  n3976 = String Length(string=w5304) -> (length=w5303:i32)
                  n3977 = Index Array(array=w5308) -> (element=w5307:u8)  [unwired: 1 in]
                  n3978 = Equal To 0?(x=w5303) -> (x = 0?=w5302:bool)
                  n3979 = Number To Boolean Array(number=w5307) -> (Boolean array=w5301:bool[])
                  n3980 = Reverse 1D Array(array=w5301) -> (reversed array=w5300:bool[])
                  n3981 = And(x=w5301, y=bool[] [FALSE, FALSE, FALSE, FALSE, FALSE, FALSE, TRUE, TRUE] ("Boolean array")) -> (x .and. y?=w5305:bool[])
                  n3982 = And(x=w5300, y=bool[] [FALSE, FALSE, TRUE, TRUE, TRUE, TRUE, TRUE, TRUE] ("Boolean array")) -> (x .and. y?=w5299:bool[])
                }
                n3983 = Concatenate Strings(w5255, w5253) -> (→"Read String":string)
                n3984 = while {
                  tunnel: w5247 -> [w5296] mode=indexing
                  tunnel: [w5292] -> w5250
                  i -> [w5292]
                  stop <- w5293 stop-if-true
                  n3985 = Search 1D Array(1D array=w5296, element=TRUE) -> (index of element=w5294:i32)  [unwired: 1 in]
                  n3986 = Less Than 0?(x=w5294) -> (x < 0?=w5293:bool)
                }
                n3987 = Delete From Array(array=w5251, length=w5250, index (row)=0) -> (array with subset deleted=w5246:bool[][])  [unwired: 1 in, 1 out]
                n3988 = Array Size(array=w5246) -> (size(s)=w5248:i32[])
                n3989 = Index Array(array=w5248) -> (element=w5240:i32)  [unwired: 1 in]
                n3990 = Greater?(x=w5240, y=w5245) -> (0:w5243:bool)
                n3991 = Subtract(x=w5240, y=w5245) -> (x-y=w5244:u32)
                n3992 = Select(t=w5244, s=w5243, f=u32 0) -> (s? t:f=w5241:u32)
                n3993 = while {
                  tunnel: w5246 -> [w5279]
                  tunnel: [w5281] -> w5239 mode=indexing
                  tunnel: w5241 -> [w5263]
                  i -> [w5280]
                  stop <- w5278 stop-if-true
                  w5270 = 6 ("index")
                  w5269 = 2 ("length")
                  # "Page 65 of \nmanual"
                  n3994 = Multiply(x=u32 3 ("y"), y=w5280) -> (x*y=w5277:u32)
                  n3995 = Divide(x=u32 102 ("y"), y=u32 65520) -> (x/y=w5287:dbl)
                  n3996 = Greater Or Equal?(x=w5277, y=w5263) -> (x >= y?=w5278:bool)
                  n3997 = Index Array(array=w5279, index (row) #1=w5277) -> (element #1=w5275:bool[], element #2=w5274:bool[], element #3=w5273:bool[])  [unwired: 5 in]
                  n3998 = Reverse 1D Array(array=w5275) -> (reversed array=w5268:bool[])
                  n3999 = Reverse 1D Array(array=w5274) -> (reversed array=w5272:bool[])
                  n4000 = Reverse 1D Array(array=w5273) -> (reversed array=w5271:bool[])
                  n4001 = Delete From Array(array=w5268, length=w5269, index=w5270) -> (array with subset deleted=w5264:bool[])  [unwired: 1 out]
                  n4002 = Delete From Array(array=w5272, length=w5269, index=w5270) -> (array with subset deleted=w5265:bool[])  [unwired: 1 out]
                  n4003 = Delete From Array(array=w5271, length=w5269, index=w5270) -> (array with subset deleted=w5266:bool[])  [unwired: 1 out]
                  n4004 = Insert Into Array(array=bool[] [] ("Boolean array"), new element #1=w5264, new element #2=w5265, new element #3=w5266) -> (w5267:bool[])  [unwired: 1 in]
                  n4005 = Boolean Array To Number(Boolean array=w5267) -> (number=w5276:u32)
                  n4006 = Multiply(x=w5287, y=w5276) -> (x*y=w5286:dbl)
                  n4007 = Decrement(x=w5286) -> (x-1=w5285:dbl)
                  n4008 = Divide(x=w5285, y=u32 100) -> (x/y=w5283:dbl)
                  n4009 = Multiply(x=w5283, y=u32 10) -> (x*y=w5281:dbl)
                }
                n4010 = Delete From Array(array=w5239) -> (array with subset deleted=w5238:dbl[])  [unwired: 2 in, 1 out]
                "Waveform Graph 5" <- w5238
                "Waveform Chart 3" <- w5238
                n4011 = call-poly <vilib>:"Mean.vi"("X"=w5238) -> ("mean"=w5237:dbl)  [unwired: 1 out]
                n4012 = case shown="True" {
                  selector: _ -> [_ _]
                  tunnel: w5237 -> [_ w5262]
                  frame False {
                  }
                  frame True {
                    n4013 = local write item#-1(FALSE ("Zero 4")) -> ()
                    "z_measure" <- w5262
                  }
                }
              }
            }
            n4014 = local read item#-1() -> (w5177)
            n4015 = local read item#-1() -> (w5176)
            n4016 = local read item#-1() -> (w5178)
            n4017 = local read item#-1() -> (w5175)
            n4018 = case shown="True" w5173 {
              tunnel: w5177 -> [_ w5205]
              tunnel: w5178 -> [_ w5204]
              frame False {
              }
              frame True {
                n4019 = Build Array(w5205, w5204) -> (w5203:void[])
                n4020 = local read item#-1() -> (w5208)
                n4021 = Build Array (concatenate)(w5208, w5203) -> (w5206:void[])
                n4022 = local write item#-1(w5206) -> ()
                n4023 = local write item#-1(FALSE ("Boolean 8")) -> ()
              }
            }
            n4024 = call "Build XY Graph"("Enable"=w5175, "Reset"=w5176, "Y Input"=w5178, "X Input"=w5177) -> ("XY Graph"=w5174:cluster{"Y":dbl[], "Y":dbl[]}[])  [unwired: 6 in, 1 out]
            n4025 = case shown="True" {
              selector: _ -> [_ _]
              frame False {
              }
              frame True {
                n4026 = local read item#-1() -> (w5209)
                n4027 = Index Array(array=w5209, index (col) #1=0 ("disabled index (col)"), index (col) #2=1 ("index (col)")) -> (element #1=w5211, element #2=w5210)  [unwired: 2 in]
                n4028 = call <vilib>:"Linear Fit.vi"("Y"=w5211, "X"=w5210) -> ()  [unwired: 9 in, 5 out]
                n4029 = local write item#-1(FALSE ("Boolean 9")) -> ()
              }
            }
            n4030 = case shown="True" {
              selector: _ -> [_ _]
              frame False {
              }
              frame True {
                n4031 = local write item#-1(dbl[][] [] ("Captured Values")) -> ()
                n4032 = local write item#-1(FALSE ("Boolean 7")) -> ()
              }
            }
            n4033 = Concatenate Strings("\r", "\n") -> (w5188:string, w5187:string)
            n4034 = case shown="True" w5179 {
              tunnel: w5186 -> [w5218 w5224]
              tunnel: w5185 -> [w5217 w5223]
              tunnel: [w5218 w5222] -> w5184
              tunnel: [w5217 w5221] -> w5183
              tunnel: w5188 -> [_ w5220]
              frame False {
              }
              frame True {
